vi "Scripting_OpenViRef.vi"(8 "error in":errorcluster, 10 "ViPath/ViName":variant, 11 "AppRef":refnum<vi>) -> (0 "error out":errorcluster, 3 "vi reference":refnum<vi>)   [LabVIEW 2012]
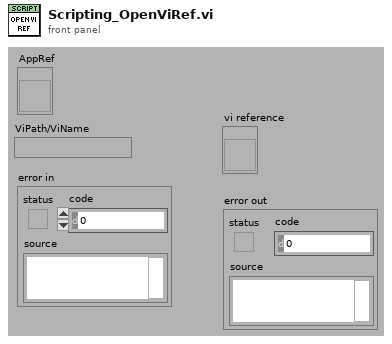
[diagram p1: front panel]
types:
  T1 = enum32{"invalid lock state", "Not Locked", "Locked (No Password)", "Password-protected"}
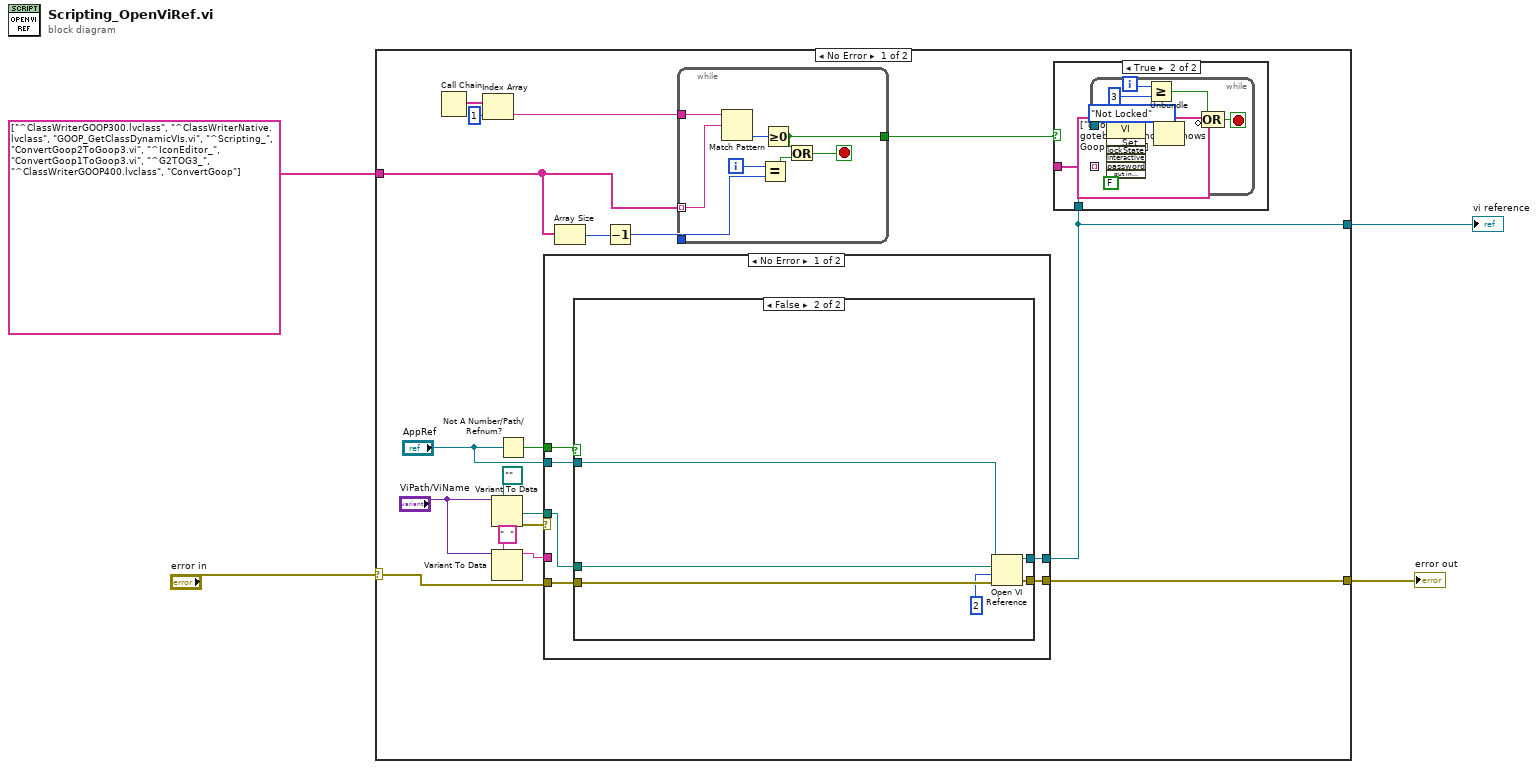
[diagram p0: block diagram]
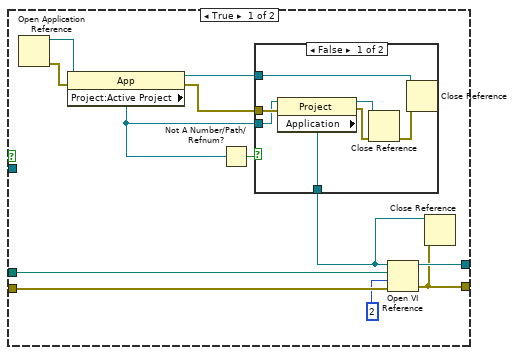
[diagram p3: hidden frame]
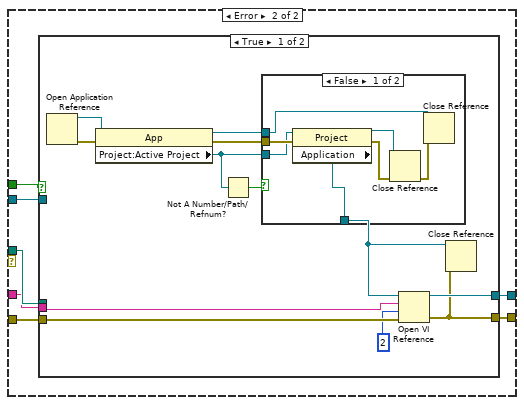
[diagram p5: hidden frame]
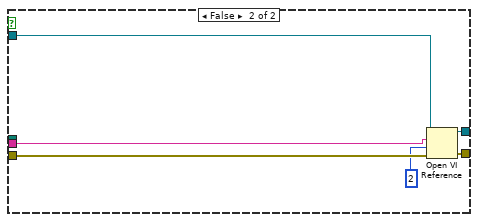
[diagram p7: hidden frame]
diagram:
  n1 = case shown="No Error" "error in" {
    selector: "error in" -> [w13 w109]
    tunnel: [w23 w109] -> w4
    tunnel: [w22 _] -> w3
    tunnel: string[] ["^ClassWriterGOOP300.lvclass", "^ClassWriterNative.lvclass", "GOOP_GetClassDynamicVIs.vi", "^Scripting_", "ConvertGoop2ToGoop3.vi", "^IconEditor_", "ConvertGoop1ToGoop3.vi", "^G2TOG3_", "^ClassWriterGOOP400.lvclass", "ConvertGoop"] -> [w5 _]
    frame No Error {
      n2 = Call Chain() -> (call chain=w12:string[])
      n3 = Index Array(array=w12, index=1) -> (element=w10:string)
      n4 = Variant To Data(type=path "" ("vi path"), Variant="ViPath/ViName") -> (data=w20:path, error out=w19:errorcluster)  [unwired: 1 in]
      n5 = Variant To Data(type="  ", Variant="ViPath/ViName") -> (data=w14:string)  [unwired: 1 in, 1 out]
      n6 = Not A Number/Path/Refnum?(number/path/refnum="AppRef") -> (NaN/Path/Refnum?=w18:bool)
      n7 = case shown="No Error" w19 {
        tunnel: w13 -> [w49 w82]
        tunnel: [w48 w81] -> w23
        tunnel: [w47 w80] -> w22
        tunnel: w20 -> [w46 w79]
        tunnel: w18 -> [w45 w78]
        tunnel: "AppRef" -> [w44 w77]
        tunnel: w14 -> [_ w76]
        frame No Error {
          n8 = case shown="False" w45 {
            tunnel: w49 -> [w61 w75]
            tunnel: [w55 w74] -> w48
            tunnel: [w56 w73] -> w47
            tunnel: w46 -> [w59 w71]
            tunnel: w44 -> [_ w70]
            frame True {
              n9 = Open Application Reference() -> (0:w57:errorcluster, 3:w58:refnum<vi>)  [unwired: 4 in]
              n10 = property class="App"(reference=w58, error in=w57) -> (reference out=w50:refnum<vi>, error out=w51:errorcluster, "Project:Active Project"=w52:refnum<vi>)
              n11 = Not A Number/Path/Refnum?(number/path/refnum=w52) -> (NaN/Path/Refnum?=w54:bool)
              n12 = case shown="False" w54 {
                tunnel: w51 -> [w68 _]
                tunnel: [w67 w69] -> w53
                tunnel: w52 -> [w66 _]
                tunnel: w50 -> [w65 w69]
                frame False {
                  n13 = property class="Project"(reference=w66, error in=w68) -> (reference out=w62:refnum<vi>, error out=w64:errorcluster, "Application"=w67:refnum<vi>)
                  n14 = Close Reference(reference=w62, error in (no error)=w64) -> (error out=w63:errorcluster)
                  n15 = Close Reference(reference=w65, error in (no error)=w63) -> ()  [unwired: 1 out]
                }
                frame True {
                }
              }
              n16 = Open VI Reference(application reference (local)=w53, vi path=w59, options=2, error in (no error)=w61) -> (vi reference=w56:refnum<vi>, error out=w55:errorcluster)  [unwired: 2 in]
              n17 = Close Reference(reference=w53, error in (no error)=w55) -> ()  [unwired: 1 out]
            }
            frame False {
              n18 = Open VI Reference(application reference (local)=w70, vi path=w71, options=2, error in (no error)=w75) -> (vi reference=w73:refnum<vi>, error out=w74:errorcluster)  [unwired: 2 in]
            }
          }
        }
        frame Error {
          n19 = case shown="True" w78 {
            tunnel: w82 -> [w94 w108]
            tunnel: [w86 w107] -> w81
            tunnel: [w93 w106] -> w80
            tunnel: w79 -> [_ _]
            tunnel: w77 -> [_ w104]
            tunnel: w76 -> [w91 w103]
            frame True {
              n20 = Open Application Reference() -> (0:w87:errorcluster, 3:w88:refnum<vi>)  [unwired: 4 in]
              n21 = property class="App"(reference=w88, error in=w87) -> (reference out=w90:refnum<vi>, error out=w89:errorcluster, "Project:Active Project"=w84:refnum<vi>)
              n22 = Not A Number/Path/Refnum?(number/path/refnum=w84) -> (NaN/Path/Refnum?=w83:bool)
              n23 = case shown="False" w83 {
                tunnel: w90 -> [w101 w102]
                tunnel: w89 -> [w100 _]
                tunnel: [w99 w102] -> w85
                tunnel: w84 -> [w98 _]
                frame False {
                  n24 = property class="Project"(reference=w98, error in=w100) -> (reference out=w95:refnum<vi>, error out=w97:errorcluster, "Application"=w99:refnum<vi>)
                  n25 = Close Reference(reference=w95, error in (no error)=w97) -> (error out=w96:errorcluster)
                  n26 = Close Reference(reference=w101, error in (no error)=w96) -> ()  [unwired: 1 out]
                }
                frame True {
                }
              }
              n27 = Open VI Reference(application reference (local)=w85, vi path=w91, options=2, error in (no error)=w94) -> (vi reference=w93:refnum<vi>, error out=w86:errorcluster)  [unwired: 2 in]
              n28 = Close Reference(reference=w85, error in (no error)=w86) -> ()  [unwired: 1 out]
            }
            frame False {
              n29 = Open VI Reference(application reference (local)=w104, vi path=w103, options=2, error in (no error)=w108) -> (vi reference=w106:refnum<vi>, error out=w107:errorcluster)  [unwired: 2 in]
            }
          }
        }
      }
      n30 = Array Size(array=w5) -> (size(s)=w8:i32)
      n31 = Decrement(x=w8) -> (x-1=w7:i32)
      n32 = while {
        tunnel: w10 -> [w43]
        tunnel: w5 -> [w42] mode=indexing
        tunnel: [w37] -> w9
        tunnel: w7 -> [w36]
        i -> [w40]
        stop <- w38 stop-if-true
        n33 = Match Pattern(string=w43, regular expression=w42) -> (offset past match=w41:i32)  [unwired: 1 in, 3 out]
        n34 = Equal?(x=w40, y=w36) -> (x = y?=w39:bool)
        n35 = Greater Or Equal To 0?(x=w41) -> (x >= 0?=w37:bool)
        n36 = Or(x=w37, y=w39) -> (x .or. y?=w38:bool)
      }
      n37 = case shown="True" w9 {
        tunnel: w22 -> [_ w25]
        tunnel: string[] ["goop rules", "i love goteborg", "Endevo Knows Goop!", "kiss"] -> [_ w24]
        frame False {
        }
        frame True {
          n38 = while {
            tunnel: w25 -> [w33]
            tunnel: w24 -> [w32] mode=indexing
            i -> [w29]
            stop <- w30 stop-if-true
            w34 = FALSE ("Interactive")
            n39 = invoke class="VI" method="Lock State.Set"(reference=w33, "lockState"=T1."Not Locked" ("Lock State"), "interactive"=w34, "password"=w32, "put in Cache"=w34) -> (error out=w31:errorcluster)  [unwired: 2 in, 6 out]
            n40 = Greater Or Equal?(x=w29, y=3) -> (x >= y?=w28:bool)
            n41 = Unbundle(w31) -> ("status"=w26:bool)  [unwired: 2 out]
            n42 = Compound Arithmetic op=OR(w28, invert w26) -> (w30:bool)
          }
        }
      }
    }
    frame Error {
    }
  }
  "vi reference" <- w3
  "error out" <- w4
